vi "Configure Voltage Limits.vi"(0 "VISA resource name":refnum<visa-resource-name>, 5 "Voltage Low Limit (0 V)":dbl min=0.0 max=400.0 format="%.1f", 7 "Voltage High Limit (300 V)":dbl=300.0 min=0.0 max=400.0 format="%.1f", 11 "error in (no error)":errorcluster) -> (4 "VISA resource name out":refnum<visa-resource-name>, 15 "error out":errorcluster)   [LabVIEW 2020, in "eec 6700.lvlib"]
doc: "Configures the <B>Voltage limit</B> in the power source instrument\n\n<B>Range</B>\n<B>For AC</B>: 0.0~300.0 V\n\nIf the output voltage is below the low limit or above the high limit of range, then the instrument will fail the test.\n\nThe Voltage Low-Limit configures a minimum voltage threshold or floor level when programming the output voltage in the testing parameters screen.\n\nThe Voltage High-Limit configures a maximum voltage threshold or ceiling level when programming the output voltage in the testing parameters screen."
uses:
  <instrlib>/eec 6700/eec 6700.lvlib
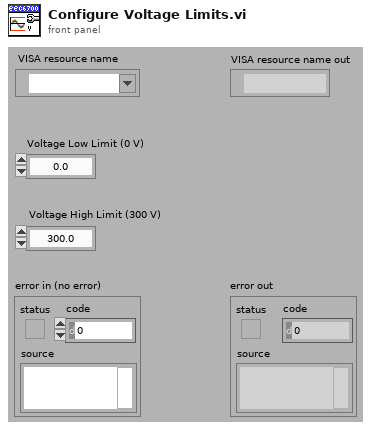
[diagram p1: front panel]
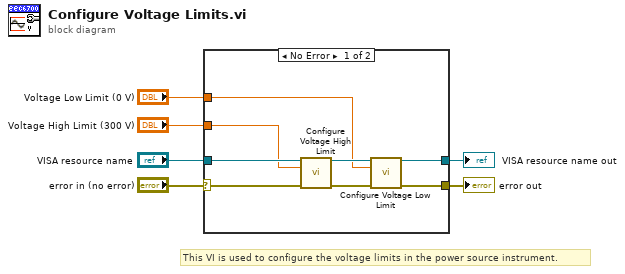
[diagram p0: block diagram]
diagram:
  # "This VI is used to configure the voltage limits in the power source instrument."
  n1 = case shown="No Error" "error in (no error)" {
    selector: "error in (no error)" -> [w9 w15]
    tunnel: "VISA resource name" -> [w14 w16]
    tunnel: [w13 w16] -> w5
    tunnel: [w12 w15] -> w4
    tunnel: "Voltage High Limit (300 V)" -> [w8 _]
    tunnel: "Voltage Low Limit (0 V)" -> [w7 _]
    frame No Error {
      n2 = call <instrlib>:"Configure Voltage High Limit.vi"("VISA resource name"=w14, "Voltage High Limit (300 V)"=w8, "error in (no error)"=w9) -> ("VISA resource name out"=w11:refnum<visa-resource-name>, "error out"=w10:errorcluster)  [unwired: 11 in]
      n3 = call <instrlib>:"Configure Voltage Low Limit.vi"("VISA resource name"=w11, "Voltage Low Limit (0 V)"=w7, "error in (no error)"=w10) -> ("VISA resource name out"=w13:refnum<visa-resource-name>, "error out"=w12:errorcluster)  [unwired: 11 in]
    }
    frame Error {
    }
  }
  "error out" <- w4
  "VISA resource name out" <- w5
